vi "EscanearObjeto.vi"(8 "Error in":errorcluster, 9 "Sesion":T1, 10 "Imagen":T2, 11 "Ángulo por foto:":dbl=45.0) -> (0 "error out":errorcluster, 1 "Sesion Out":T1, 2 "Image":T2(plugin-control), 3 "Dimension k":u8)   [LabVIEW 2020]
doc: "Este VI escanea el objeto colocado frente a la cámara seleccionada. Un motor a pasos es activado para girar un cierto número de grador y capturar una imagen del objeto en diferentes grados de rotación hasta lograr los 360°. Cada uno de las imágenes obtenidas se introduce en el subVI Detección_ROI para calcular el recuadro mínimo en el que se puede encerrar al objeto, para sólo tomar ese recuadro de la imagen y posteriormente normalizar la imagen a un tamaño de 400x250. Cada una de estas imágenes son expresadas como un solo vector de 1x(250x400x3) (un vector para cada plano de color) y se juntan en una matriz. Para esta matriz se calcula la SVD y se selecciona sólo los primeros k vectores, de la base formada por la matriz U , que contengan más del 95% de la información de la matriz de entrada. Posteriormente, para esa base dada, se calcula para cada imagen los coeficientes de la base que expresan el punto de esa imagen en el espacio generado por la base. Por último, toda esta información es mandada y almacenada a la base de datos."
uses:
  <vilib>/vision/Image Controls.llb/IMAQ Image.ctl
  <vilib>/userdefined/High Color/IMAQdx.ctl
  <vilib>/Analysis/BLAS.llb/LV_Transpose.ctl
  <vilib>/DAQmx/write.llb/DAQmx Write (Digital 1D Bool NChan 1Samp 1Line).vi
  <vilib>/Analysis/baseanly.llb/Mean (DBL).vi
  <vilib>/DAQmx/miscellaneous.llb/DAQmx Fill In Error Info.vi
  <vilib>/Analysis/7linalg.llb/Real SVD Decomposition.vi
  <vilib>/Analysis/BLAS.llb/dgemm - General Matrix-Matrix Product (DBL).vi
  <vilib>/vision/driver/NI_Vision_Acquisition_Software.lvlib
  <vilib>/Analysis/NI_AALPro.lvlib
  <vilib>/vision/NI_Vision_Development_Module.lvlib
  <vilib>/Analysis/NI_AALBase.lvlib
  <vilib>/Analysis/NI_AALBLAS.lvlib
panel:
  # "1600x1200"
  # "para 8 fotos: 45°\npara 36 fotos: 10°\npara 72 fotos: 5°\npara 48 fotos: 7.5°"
  # "to do:\navisar que se ha escaneado y almacenado correctamente\n\nadicional: \ncambiar todo a tipo float?\nparametrizar el tamaño m del vector en toto el codigo"
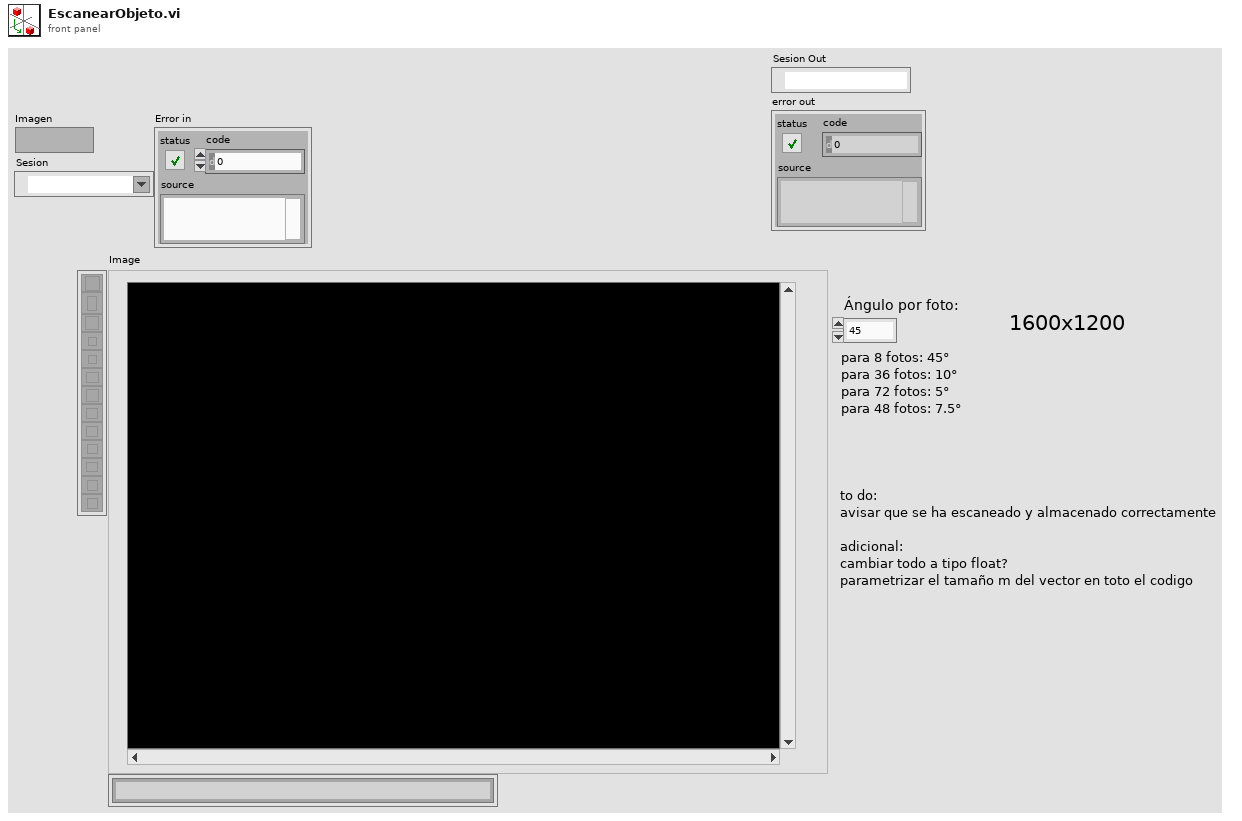
[diagram p1: front panel]
types:
  T1 = typedef "IMAQdx.ctl" = refnum<k21>
  T2 = typedef "IMAQ Image.ctl" = refnum<image>
  T3 = typedef "Image Type" = u32
  T4 = typedef "NI_AALBLAS.lvlib/LV_Transpose.ctl" = i32
  T5 = typedef "NI_Matrix.lvlib/RealMatrix.ctl" = dbl[][]
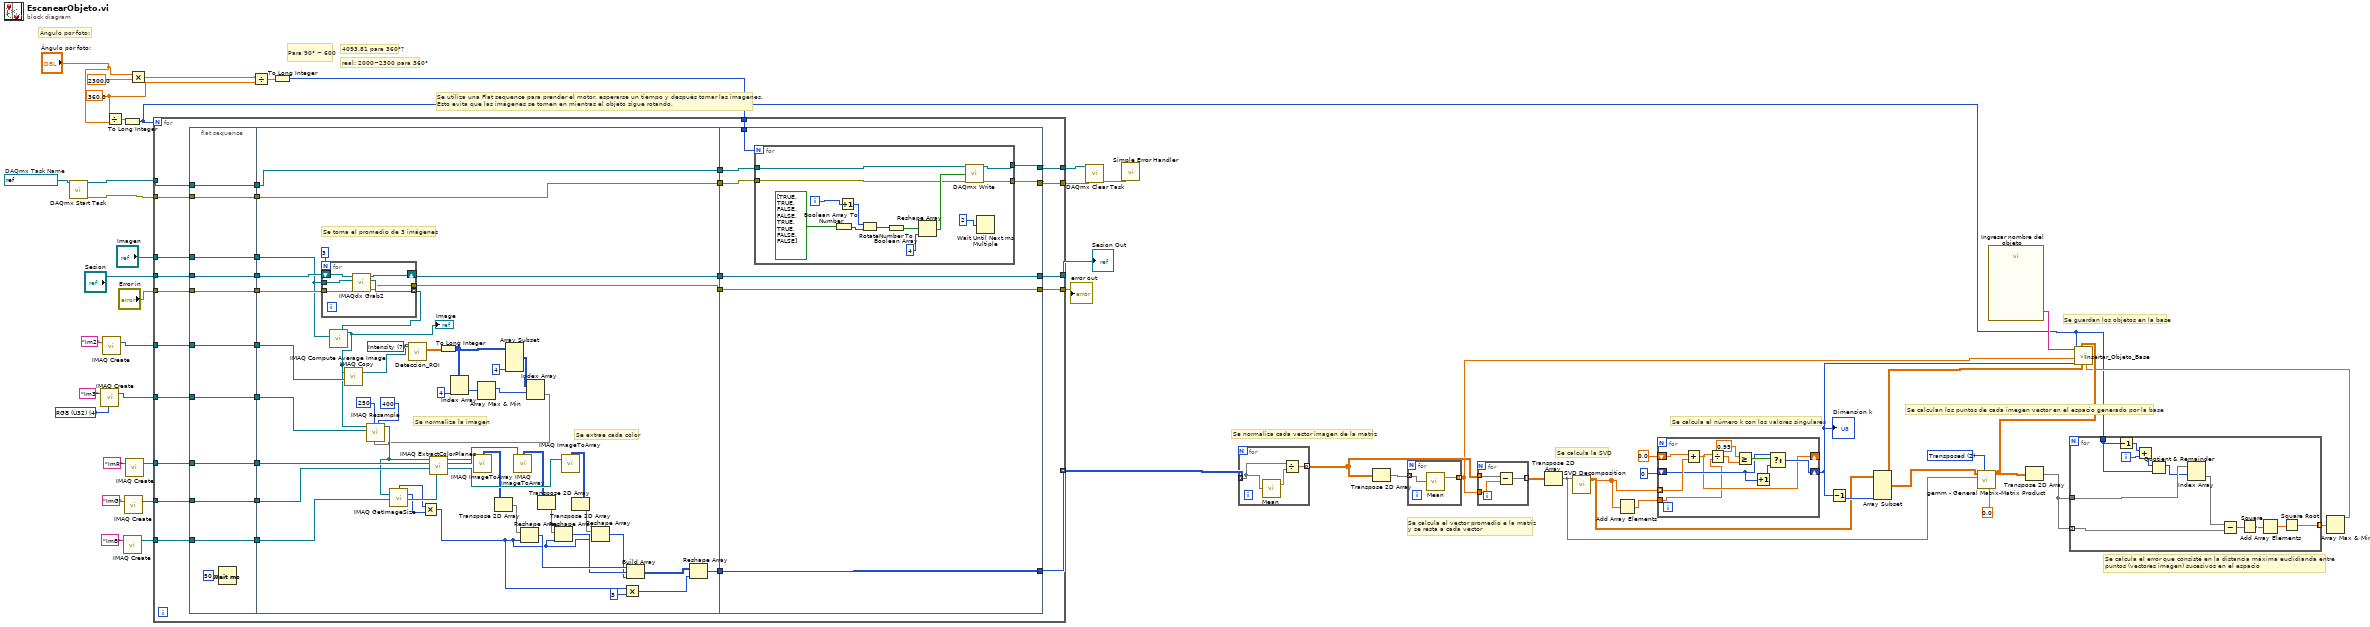
[diagram p0: block diagram]
diagram:
  w17 = refnum<k21> "MotorPasos"  # DAQmx Task Name
  w18 = 360.0 ("y")
  w24 = T3 4 items=["Grayscale (U8)", "Grayscale (I16)", "Grayscale (SGL)", "Complex (CSG)", "RGB (U32)", "HSL (U32)", "RGB (U64)", "Grayscale (U16)"] ("Image Type")
  w33 = T4 2 items=["Direct", "Conjugated & Transposed", "Transposed"] ("operation A")
  # "Se guardan los objetos en la base"
  # "Se calcula el error que consisté en la distancia máxima euclidianda entre\npuntos (vectores imagen) sucesivos en el espacio"
  # "Se calculan los puntos de cada imegen vector en el espacio generado por la base"
  # "Se calcula el número k con los valores singulares"
  # "Se calcula la SVD"
  # "Se calcula el vector promedio e la matriz\ny se resta a cada vector"
  # "Se normaliza cada vector imagen de la matriz"
  # "Se utiliza una Flat sequence para prender el motor, esperarse un tiempo y después tomar las imagenes. \nEsto evita que las imágenes se tomen en mientras el objeto sigue rotando."
  # "Ángulo por foto:"
  # "real: 2000~2300 para 360°"
  # "4093.81 para 360°?"
  # "Para 90° ~ 600"
  n1 = call <vilib>:"DAQmx Start Task.vi"("task/channels in"=w17) -> ("task out"=w16:refnum<k21>, "error out"=w15:errorcluster)  [unwired: 13 in]
  n2 = call "IMAQ Create"("Image Name"="Im3", "Image Type"=w24) -> ("New Image"=w25:T2)  [unwired: 3 in, 1 out]
  n3 = call "IMAQ Create"("Image Name"="Im2") -> ("New Image"=w28:T2)  [unwired: 4 in, 1 out]
  n4 = Divide(x=w18, y="Ángulo por foto:") -> (x/y=w20:dbl)
  n5 = To Long Integer(number=w20) -> (32bit integer=w1:i32)
  n6 = call "IMAQ Create"("Image Name"="ImB") -> ("New Image"=w42:T2)  [unwired: 4 in, 1 out]
  n7 = call "IMAQ Create"("Image Name"="ImG") -> ("New Image"=w43:T2)  [unwired: 4 in, 1 out]
  n8 = call "IMAQ Create"("Image Name"="ImR") -> ("New Image"=w44:T2)  [unwired: 4 in, 1 out]
  n9 = Multiply(x="Ángulo por foto:", y=2300.0) -> (x*y=w21:dbl)
  n10 = Divide(x=w21, y=w18) -> (x/y=w19:dbl)
  n11 = To Long Integer(number=w19) -> (32bit integer=w14:i32)
  n12 = for {
    N: w1 -> [_]
    tunnel: "Sesion" -> [w82]
    tunnel: "Error in" -> [w81]
    tunnel: "Imagen" -> [w73]
    tunnel: [w80] -> w48
    tunnel: w44 -> [w79]
    tunnel: w43 -> [w78]
    tunnel: w42 -> [w77]
    tunnel: [w76] -> w51 mode=indexing
    tunnel: w28 -> [w75]
    tunnel: w25 -> [w74]
    tunnel: w16 -> [w58]
    tunnel: w15 -> [w55]
    tunnel: w14 -> [w62]
    tunnel: [w61] -> w13
    tunnel: [w60] -> w12
    tunnel: [w52] -> w2
    n13 = flat-sequence {
      tunnel: w73 -> [w86]
      tunnel: w74 -> [w87]
      tunnel: w75 -> [w88]
      tunnel: w77 -> [w89]
      tunnel: w78 -> [w90]
      tunnel: w79 -> [w91]
      tunnel: w81 -> [w92]
      tunnel: w82 -> [w93]
      tunnel: [w93] -> w72
      tunnel: [w92] -> w71
      tunnel: [w91] -> w70
      tunnel: [w90] -> w69
      tunnel: [w89] -> w68
      tunnel: [w88] -> w67
      tunnel: [w87] -> w66
      tunnel: [w86] -> w65
      tunnel: [w84] -> w59
      tunnel: w58 -> [w84]
      tunnel: [w83] -> w56
      tunnel: w55 -> [w83]
      tunnel: w72 -> [w140]
      tunnel: w71 -> [w139]
      tunnel: w70 -> [w137]
      tunnel: w69 -> [w136]
      tunnel: w68 -> [w135]
      tunnel: w67 -> [w106]
      tunnel: w66 -> [w101]
      tunnel: w65 -> [w98]
      tunnel: [w138] -> w64
      tunnel: [w116] -> w63
      tunnel: w59 -> [w96]
      tunnel: [w96] -> w57
      tunnel: w56 -> [w95]
      tunnel: [w95] -> w54
      tunnel: [w94] -> w53
      tunnel: [w153] -> w76
      tunnel: [w154] -> w80
      tunnel: w64 -> [w154]
      tunnel: w63 -> [w153]
      tunnel: w62 -> [w152]
      tunnel: [w151] -> w61
      tunnel: [w150] -> w60
      tunnel: w57 -> [w149]
      tunnel: w54 -> [w148]
      tunnel: w53 -> [w147]
      tunnel: [w147] -> w52
      frame #0 {
        n14 = Wait (ms)(milliseconds to wait=u32 50) -> ()  [unwired: 1 out]
      }
      frame #1 {
        w115 = 7 items=["Red", "Green", "Blue", "Hue", "Saturation", "Luminance", "Value", "Intensity"] ("Color Plane (Color Plane Extraction 1)")
        # "Se extrae cada color"
        # "Se normaliza la imagen"
        # "Se toma el promedio de 3 imágenes"
        n15 = for {
          N: 3 -> [_]
          tunnel: w139 -> [w145]
          tunnel: w98 -> [w144]
          shift-right: [w143] -> w138
          shift-left: w140 -> [w146]
          tunnel: [w142] -> w99 mode=indexing
          tunnel: [w141] -> w94
          n16 = call <vilib>:"IMAQdx Grab2.vi"("error in"=w145, "Image In"=w144, "Session In"=w146) -> ("error out"=w141:errorcluster, "Image Out"=w142:T2, "Session Out"=w143:T1)  [unwired: 5 in, 1 out]
        }
        n17 = call "IMAQ Compute Average Image"("Image Dst"=w98, "Images"=w99) -> ("Image Dst Out"=w97:T2)  [unwired: 8 in, 1 out]
        "Image" <- w97
        n18 = call "IMAQ Copy"("Image Dst"=w106, "Image Src"=w97) -> ("Image Dst Out"=w107:T2)  [unwired: 4 in, 1 out]
        n19 = call "Detección_ROI.vi"("Image In"=w107, "Color Plane (Color Plane Extraction 1)"=w115) -> ("Particle Measurements (Pixels) (Particle Analysis 1)"=w114:dbl[][])  [unwired: 21 in, 4 out]
        n20 = To Long Integer(number=w114) -> (32bit integer=w112:i32[][])
        n21 = Index Array(array=w112, index (col)=4 ("disabled index (col)")) -> (element=w110:i32[])  [unwired: 1 in]
        n22 = Array Max & Min(array=w110) -> (max index (indices)=w108:i32)  [unwired: 3 out]
        n23 = Array Subset(array=w112, length (col)=4 ("length")) -> (w109:i32[][])  [unwired: 3 in]
        n24 = Index Array(array=w109, index (row)=w108) -> (element=w102:i32[])  [unwired: 1 in]
        n25 = call "IMAQ Resample"("X Resolution"=400 ("Y Resolution"), "Optional Rectangle"=w102, "Y Resolution"=250, "Image Dst"=w101, "Image Src"=w97) -> ("Image Dst Out"=w103:T2)  [unwired: 5 in, 1 out]
        n26 = call "IMAQ GetImageSize"("Image"=w103) -> ("Y Resolution"=w125:i32, "X Resolution"=w124:i32)  [unwired: 3 in, 1 out]
        n27 = Multiply(x=w124, y=w125) -> (x*y=w120:i32)
        n28 = call "IMAQ ExtractColorPlanes"("Blue or Luma or Val or Inten Plane"=w135, "Green or Sat Plane"=w136, "Red or Hue Plane"=w137, "Image Src"=w103) -> ("Blue or Luma or Val or Inten Plane out"=w133:T2, "Green or Sat Plane out"=w134:T2, "Red or Hue Plane out"=w132:T2)  [unwired: 4 in, 1 out]
        n29 = call "IMAQ ImageToArray"("Image"=w132) -> ("Image Pixels (U8)"=w131:u8[][])  [unwired: 3 in, 4 out]
        n30 = Transpose 2D Array(2D array=w131) -> (transposed array=w128:u8[][])
        n31 = call "IMAQ ImageToArray"("Image"=w134) -> ("Image Pixels (U8)"=w130:u8[][])  [unwired: 3 in, 4 out]
        n32 = Reshape Array(w128, w120) -> (w123:u8[])
        n33 = Transpose 2D Array(2D array=w130) -> (transposed array=w127:u8[][])
        n34 = Reshape Array(w127, w120) -> (w122:u8[])
        n35 = call "IMAQ ImageToArray"("Image"=w133) -> ("Image Pixels (U8)"=w129:u8[][])  [unwired: 3 in, 4 out]
        n36 = Transpose 2D Array(2D array=w129) -> (transposed array=w126:u8[][])
        n37 = Reshape Array(w126, w120) -> (w121:u8[])
        n38 = Multiply(x=w120, y=3) -> (x*y=w118:i32)
        n39 = Build Array(w123, w122, w121) -> (w117:u8[][])
        n40 = Reshape Array(w117, w118) -> (w116:u8[])
      }
      frame #2 {
        n41 = for {
          N: w152 -> [_]
          tunnel: [w159] -> w151
          tunnel: [w158] -> w150
          tunnel: w149 -> [w157]
          tunnel: w148 -> [w156]
          i -> [w155]
          n42 = Boolean Array To Number(Boolean array=bool[] [TRUE, TRUE, FALSE, FALSE, TRUE, TRUE, FALSE, FALSE] ("data")) -> (number=w162:u8)
          n43 = Increment(x=w155) -> (x+1=w160:i32)
          n44 = Rotate(1:w162, 2:w160) -> (0:w166:u8)
          n45 = Number To Boolean Array(number=w166) -> (Boolean array=w165:bool[])
          n46 = Reshape Array(w165, 4 ("dimension size")) -> (w163:bool[])
          n47 = call-poly <vilib>:"DAQmx Write.vi"("task/channels in"=w157, "data"=w163, "error in"=w156) -> ("task out"=w159:refnum<k21>, "error out"=w158:errorcluster)  [unwired: 10 in, 1 out]
          n48 = Wait Until Next ms Multiple(millisecond multiple=u32 2) -> ()  [unwired: 1 out]
        }
      }
    }
  }
  "Sesion Out" <- w48
  "error out" <- w2
  n49 = call <vilib>:"DAQmx Clear Task.vi"("task in"=w13, "error in"=w12) -> ("error out"=w3:errorcluster)  [unwired: 13 in]
  n50 = call <vilib>:"Simple Error Handler.vi"("error in (no error)"=w3) -> ()  [unwired: 4 in, 5 out]
  n51 = for {
    tunnel: [w170] -> w30 mode=indexing
    tunnel: w51 -> [w168] mode=indexing
    n52 = call-poly <vilib>:"Mean.vi"("X"=w168) -> ("mean"=w169:dbl)  [unwired: 1 out]
    n53 = Divide(x=w168, y=w169) -> (x/y=w170:dbl[])
  }
  n54 = Transpose 2D Array(2D array=w30) -> (transposed array=w35:dbl[][])
  n55 = for {
    tunnel: w35 -> [w172] mode=indexing
    tunnel: [w171] -> w29 mode=indexing
    n56 = call-poly <vilib>:"Mean.vi"("X"=w172) -> ("mean"=w171:dbl)  [unwired: 1 out]
  }
  n57 = for {
    tunnel: [w175] -> w36 mode=indexing
    tunnel: w29 -> [w174]
    tunnel: w30 -> [w173] mode=indexing
    n58 = Subtract(x=w173, y=w174) -> (x-y=w175:dbl[])
  }
  n59 = Transpose 2D Array(2D array=w36) -> (transposed array=w41:dbl[][])
  n60 = call-poly <vilib>:"SVD Decomposition.vi"("A"=w41) -> ("Matrix U"=w39:T5, "Vector S"=w37:dbl[])  [unwired: 6 in, 3 out]
  n61 = Add Array Elements(numeric array=w37) -> (sum=w38:dbl)
  n62 = for {
    tunnel: w37 -> [w184] mode=indexing
    shift-right: [w180] -> w49
    shift-left: u8 0 -> [w179]
    shift-right: [w177] -> _
    shift-left: 0.0 -> [w185]
    tunnel: w38 -> [w176]
    n63 = Add(x=w185, y=w184) -> (x+y=w177:dbl)
    n64 = Divide(x=w177, y=w176) -> (x/y=w183:dbl)
    n65 = Greater Or Equal?(x=0.95, y=w183) -> (x >= y?=w181:bool)
    n66 = Increment(x=w179) -> (x+1=w178:u8)
    n67 = Select(t=w179, s=w181, f=w178) -> (s? t:f=w180:u8)
  }
  "Dimension k" <- w49
  n68 = Decrement(x=w49) -> (x-1=w40:u8)
  n69 = Array Subset(array=w39, length (col)=w40) -> (w50:T5)  [unwired: 3 in]
  n70 = call-poly <vilib>:"gemm - General Matrix-Matrix Product.vi"("beta"=0.0, "operation A"=w33, "B"=w41, "A"=w50) -> ("dgemm"=w10:T5)  [unwired: 6 in, 1 out]
  n71 = call "Ingresar nombre del objeto"() -> ("Objeto"=w23:string)  [unwired: 17 in, 2 out]
  n72 = Transpose 2D Array(2D array=w10) -> (transposed array=w9:T5)
  n73 = for {
    tunnel: w9 -> [w191] mode=indexing
    tunnel: w9 -> [w193]
    tunnel: w1 -> [w197]
    tunnel: [w186] -> w8 mode=indexing
    i -> [w196]
    n74 = Decrement(x=w197) -> (x-1=w195:i32)
    n75 = Add(x=w195, y=w196) -> (x+y=w194:i32)
    n76 = Quotient & Remainder(x=w194, y=w197) -> (x-y*floor(x/y)=w192:i32)  [unwired: 1 out]
    n77 = Index Array(array=w193, index (row)=w192) -> (element=w190:dbl[])  [unwired: 1 in]
    n78 = Subtract(x=w190, y=w191) -> (x-y=w189:dbl[])
    n79 = Square(x=w189) -> (x^2=w188:dbl[])
    n80 = Add Array Elements(numeric array=w188) -> (sum=w187:dbl)
    n81 = Square Root(x=w187) -> (sqrt(x)=w186:dbl)
  }
  n82 = Array Max & Min(array=w8) -> (max value=w7:dbl)  [unwired: 3 out]
  n83 = call "Insertar_Objeto_Base.vi"("Error"=w7, "Base"=w50, "Puntos Fotos"=w10, "Dimensión k del espacio"=w49, "Vector promedio c"=w29, "# Fotos"=w1, "Nombre del objeto"=w23) -> ()  [unwired: 5 in]
